vi "Reset Usage.vi"(7 "Pump ID (0:A)":T1, 8 "error in (no error)":errorcluster, 11 "VISA resource in":refnum<visa-resource-name>) -> (0 "error out":errorcluster, 3 "VISA resource out":refnum<visa-resource-name>)   [LabVIEW 2015, in "Global FIA milliGAT.lvlib"]
doc: "Resets the total volume that the pump has pumped to zero."
uses:
  Global FIA milliGAT.lvlib
  Private/Pump Parameter.ctl
  Pump Address.ctl
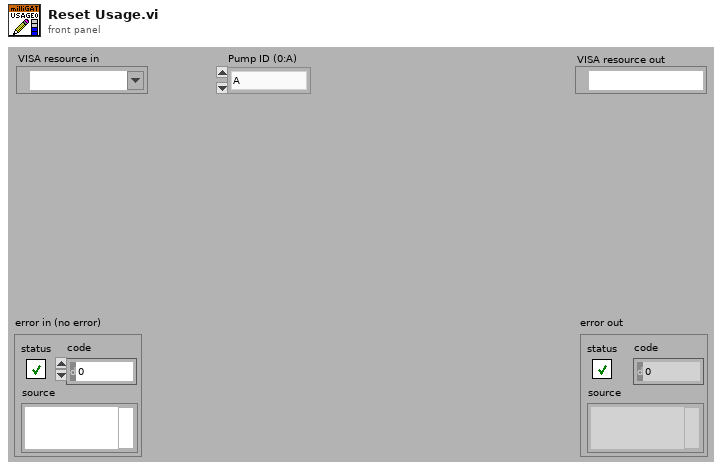
[diagram p1: front panel]
types:
  T1 = typedef "Global FIA milliGAT.lvlib/Pump Address.ctl" = enum16{"A", "B", "C", "D", "E", "F", "G", "H", "I", "J", "K", "L", "M", "N", "O", "P", "Q", "R", "S", "T", "U", "V", "W", "X", "Y", "Z", "a", "b", "c", "d", "e", "f", "g", "h", "i", "j", "k", "l", "m", "n", "o", "p", "q", "r", "s", "t", "u", "v", "w", "x", "y", "z", "0", "1", "2", "3", "4", "5", "6", "7", "8", "9"}
  T2 = typedef "Global FIA milliGAT.lvlib/Pump Parameter.ctl" = enum16{"Enabled", "EU", "EU Calibration Factor", "Fixed Asp or Disp", "Starting Position", "Starting Flow", "Peak Flow", "Flow Acceleration", "Flow Deceleration", "Session Volume", "Max Pressure", "Backlash (usteps)", "BL Calibration Factor", "BL Correction Enabled", "Min Flow", "Max Flow", "Min Acceleration", "Max Acceleration", "Service Volume", "Life Volume"}
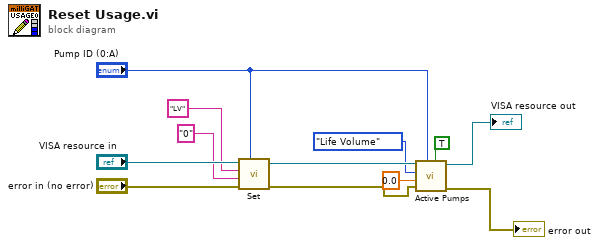
[diagram p0: block diagram]
diagram:
  n1 = call "Set.vi"("Pump ID (0:A)"="Pump ID (0:A)", "error in (no error)"="error in (no error)", "Expression"="0", "Parameter"="LV" ("Parameter Name"), "VISA resource in"="VISA resource in") -> ("error out"=w1:errorcluster, "VISA resource out"=w8:refnum<visa-resource-name>)  [unwired: 5 in]
  n2 = call "Active Pumps.vi"("Action (F:Read)"=TRUE, "Pump ID (0:A)"="Pump ID (0:A)", "error in (no error)"=w1, "Value in"=0.0, "Parameter"=Pump_Parameter."Life Volume", "VISA resource in"=w8) -> ("error out"=→"error out":errorcluster, "VISA resource out"=→"VISA resource out":refnum<visa-resource-name>)  [unwired: 2 in, 2 out]
